vi "IQA.vi"() -> ()   [LabVIEW 2017]
uses:
  Sub VIs/Control/State machine.ctl
  <vilib>/Utility/miscctls.llb/LVPointTypeDef.ctl
  <vilib>/addons/database/Connection.llb/Conn ObjectReference.ctl
  5081ad37-31e8-4bc8-bbee-fac5e5d8bad7.vi
  <vilib>/Array/Sort 2D Array - Pop Stack.vi
  <vilib>/Array/Sort 2D Array - Push Stack.vi
  <vilib>/addons/database/Connection.llb/DB Tools Open Connec (Path).vi
  <vilib>/addons/database/Connection.llb/Conn Execute.vi
  <vilib>/addons/database/Recordset.llb/Rec Fetch Recordset Data (R).vi
  <vilib>/addons/database/Recordset.llb/Rec Destroy - Connection.vi
  <vilib>/addons/database/_DB Variant To Data/Database Variant To Data.xnode
  <vilib>/Utility/config.llb/NI_LVConfig.lvlib
  <vilib>/addons/database/NI_Database_API.lvlib
panel:
  out "local":T1
  out "server":T1
  in  "Search":string(combo)
  in  "IQA Check":bool
  in  "Refresh":bool
  in  "Invoice CODE":string(combo)
  out "Invoice Date":timestamp format="%<%d/%m/%Y>T"
  out "Table":string[][](table)
  # "IQA HISTORY"
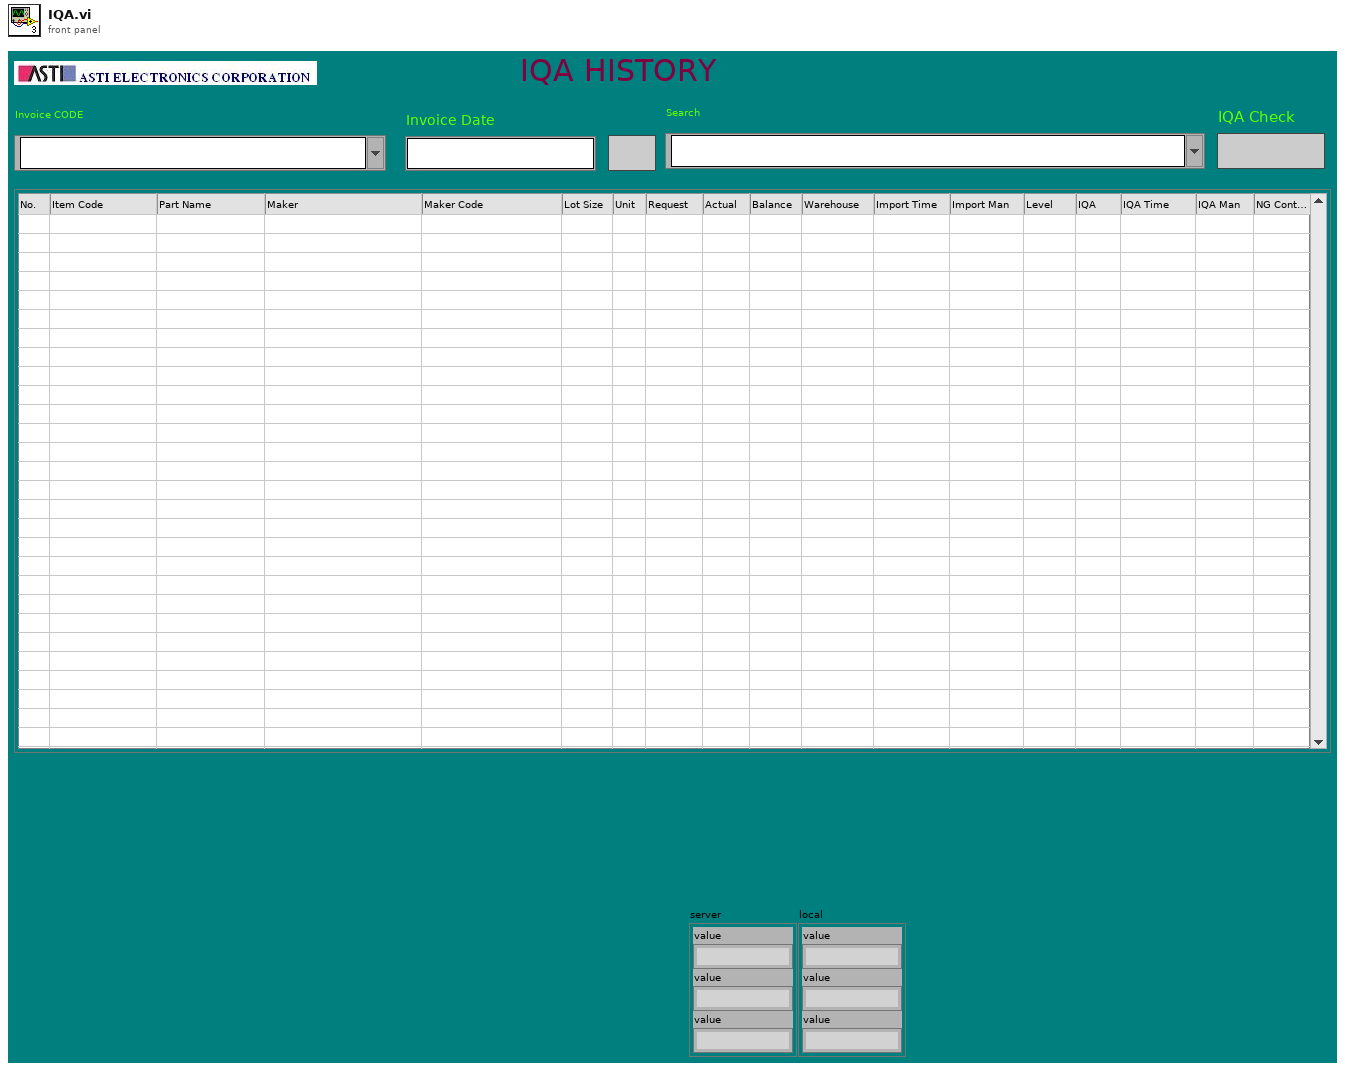
[diagram p1: front panel]
types:
  T1 = cluster{"value":string, "value":string, "value":string}
  T2 = typedef "NI_Database_API.lvlib/Conn ObjectReference.ctl" = refnum<k1>
  T3 = typedef "LVPointTypeDef.ctl" = cluster{"Horizontal":i16, "Vertical":i16}
  T4 = typedef "State machine.ctl" = enum16{"Licence check", "Initial", "Log in", "Creat Config file", "Network setting", "Creat database 1", "Creat database 2", "Creat database 3", "Transfer", "Begin", "Exit"}
  T5 = typedef "NI_LVConfig.lvlib/Config Data RefNum.ctl" = refnum<k1>
  T6 = typedef "NI_Database_API.lvlib/Rec ObjectReference.ctl" = refnum<k1>
  T7 = cluster{"[0]":string, "[1]":string, "[2]":string, "[3]":string, "[4]":string, "[5]":string, "[6]":string, "[7]":string, "[8]":string, "[9]":string, "[10]":string, "[11]":string, "[12]":string, "[13]":string, "[14]":string, "[15]":string}
  T8 = cluster{"[0]":string, "[1]":string, "[2]":string, "[3]":string, "[4]":string, "[5]":string, "[6]":string, "[7]":string, "[8]":string, "[9]":string, "[10]":string, "[11]":string, "[12]":string, "[13]":string, "[14]":string, "[15]":string}[]
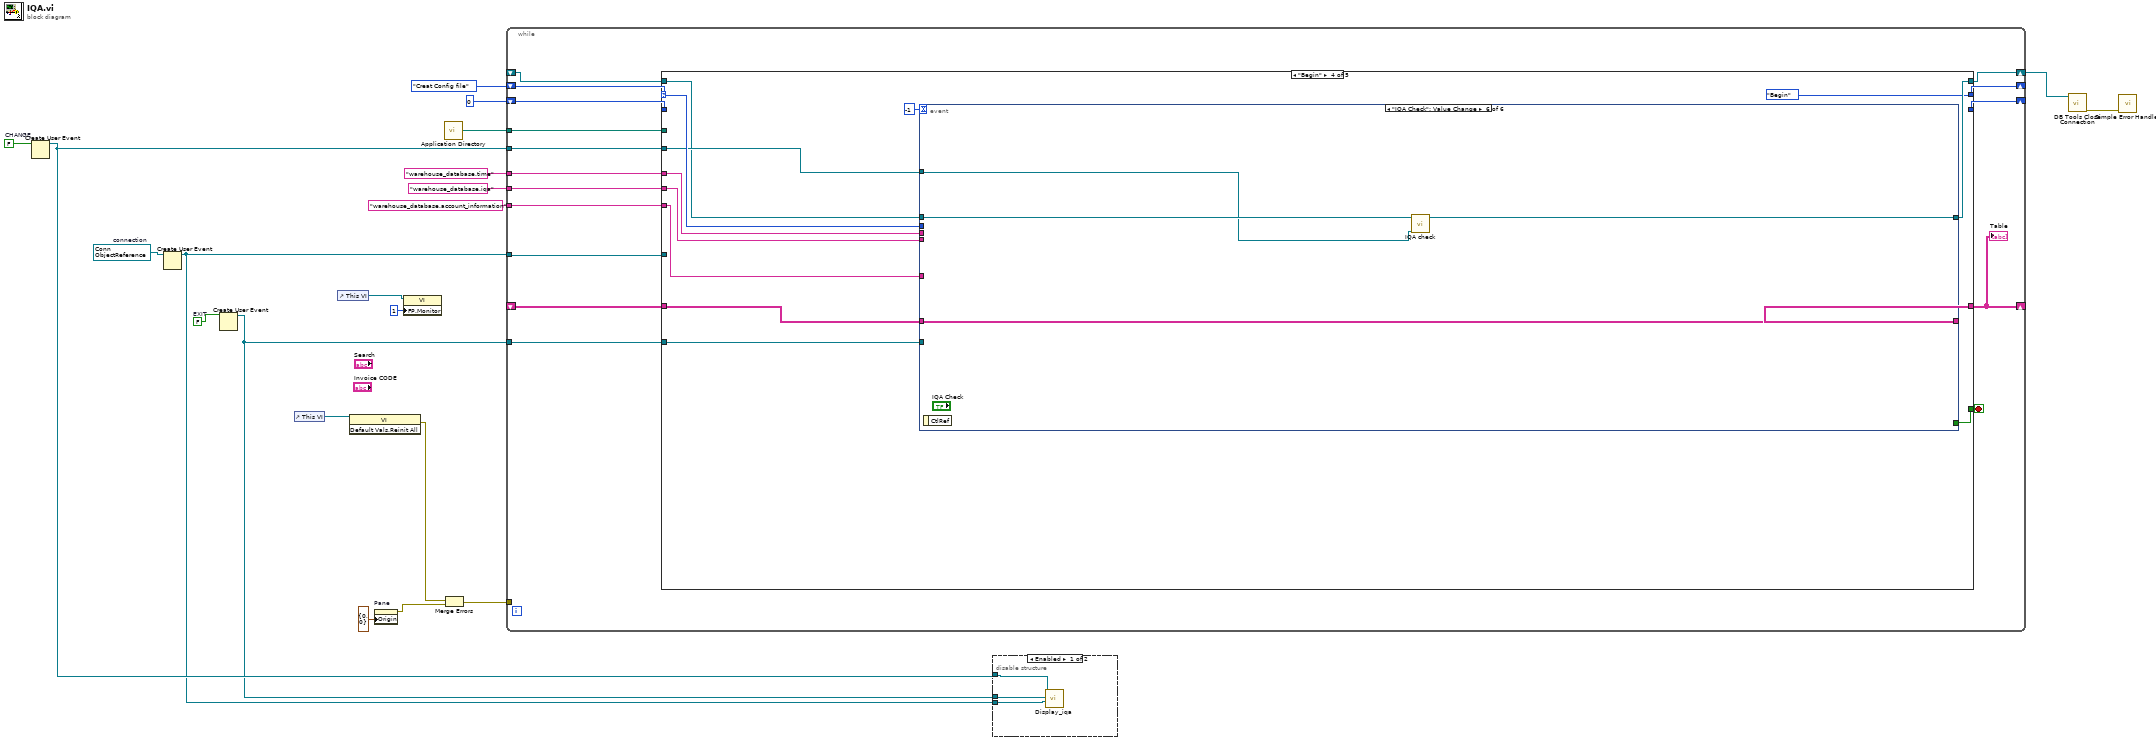
[diagram p0: block diagram]
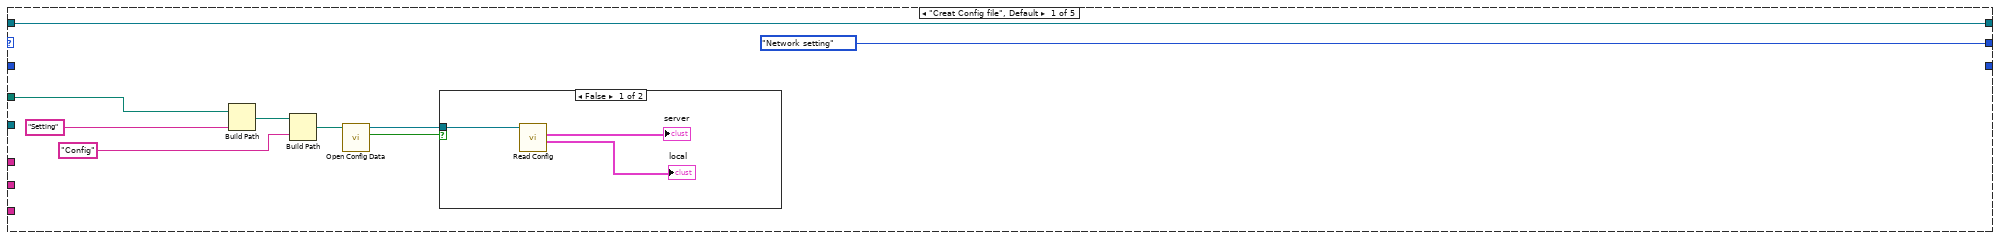
[diagram p3: hidden frame]
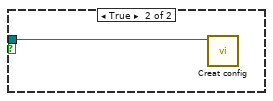
[diagram p4: hidden frame]
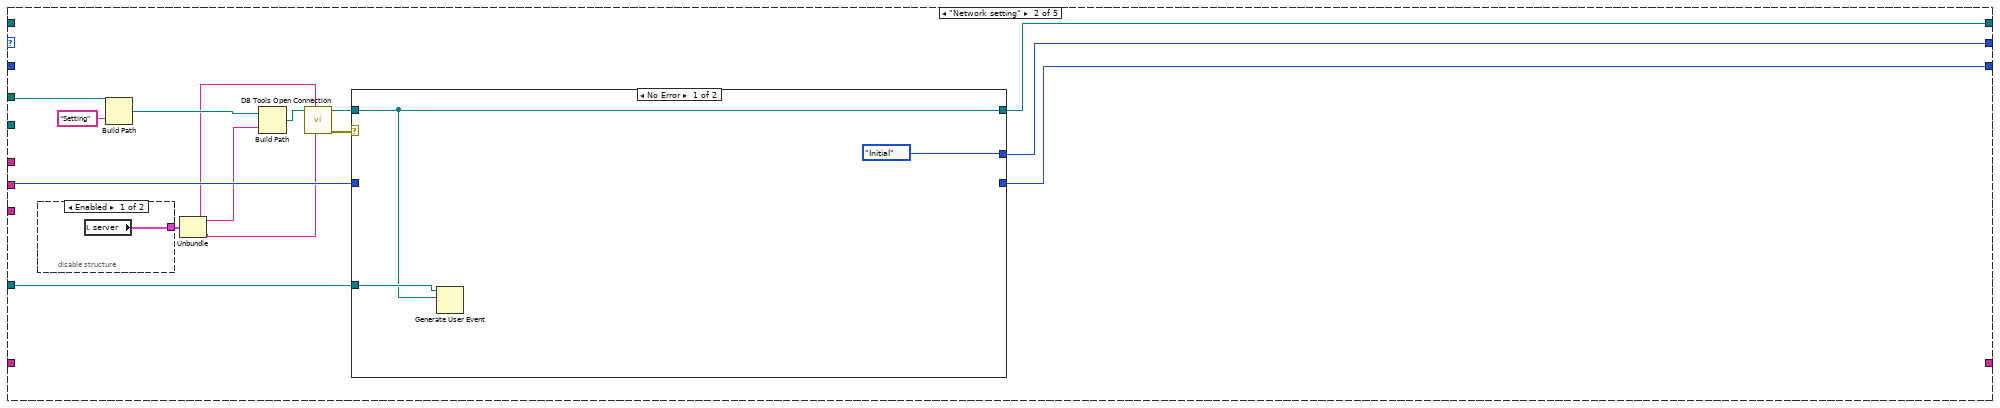
[diagram p5: hidden frame]
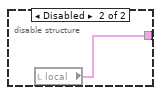
[diagram p6: hidden frame]
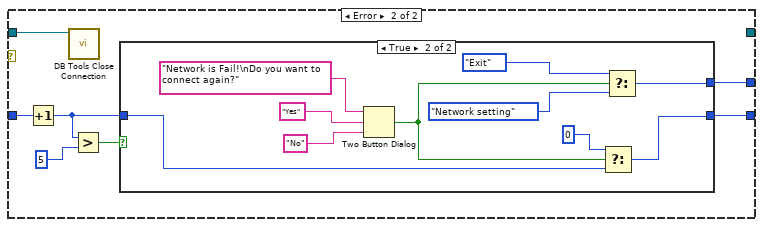
[diagram p7: hidden frame]
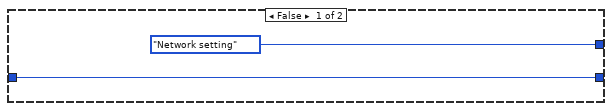
[diagram p8: hidden frame]
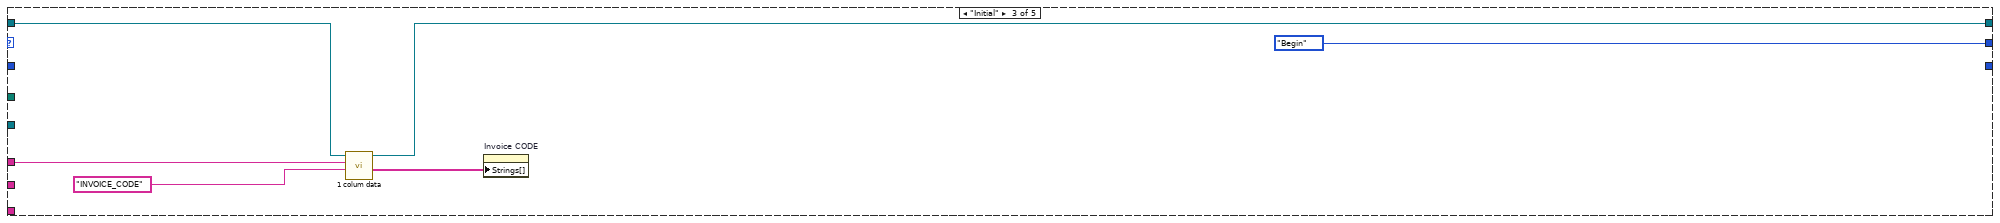
[diagram p9: hidden frame]
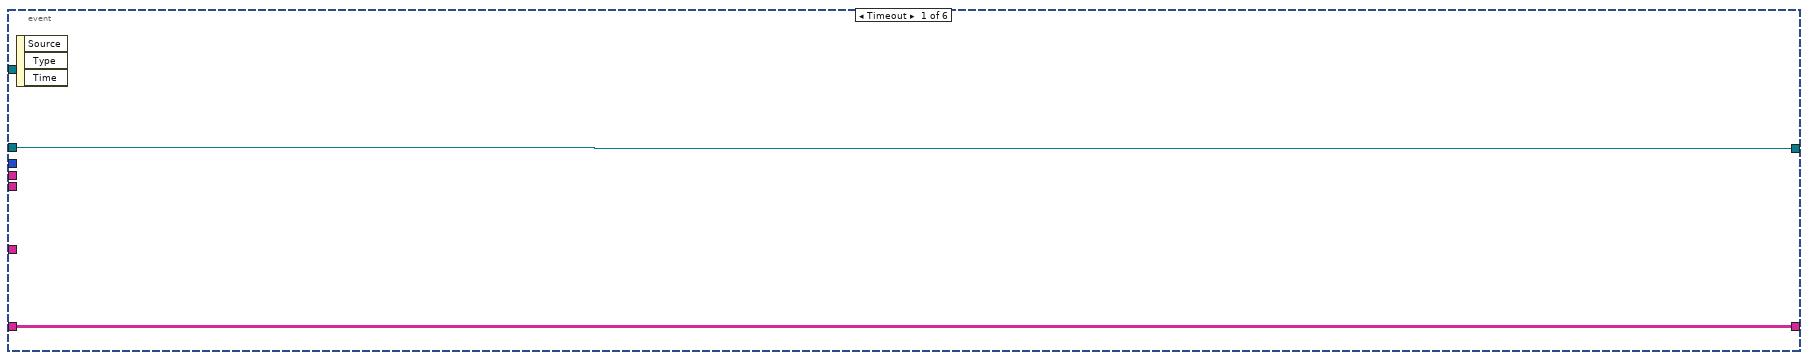
[diagram p10: hidden frame]
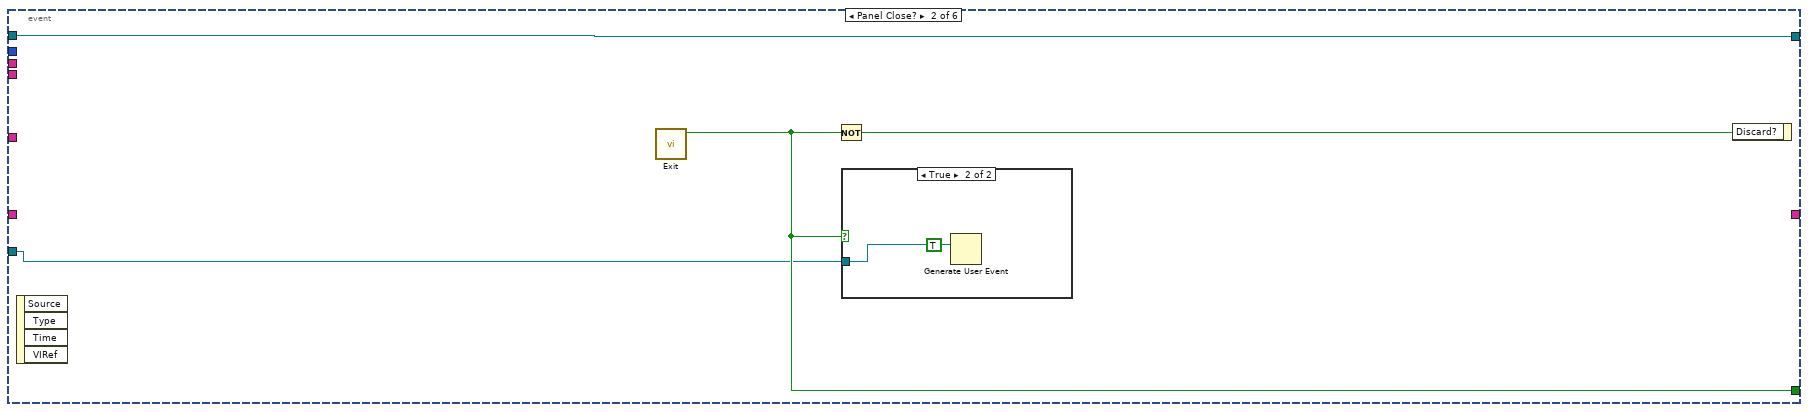
[diagram p11: hidden frame]
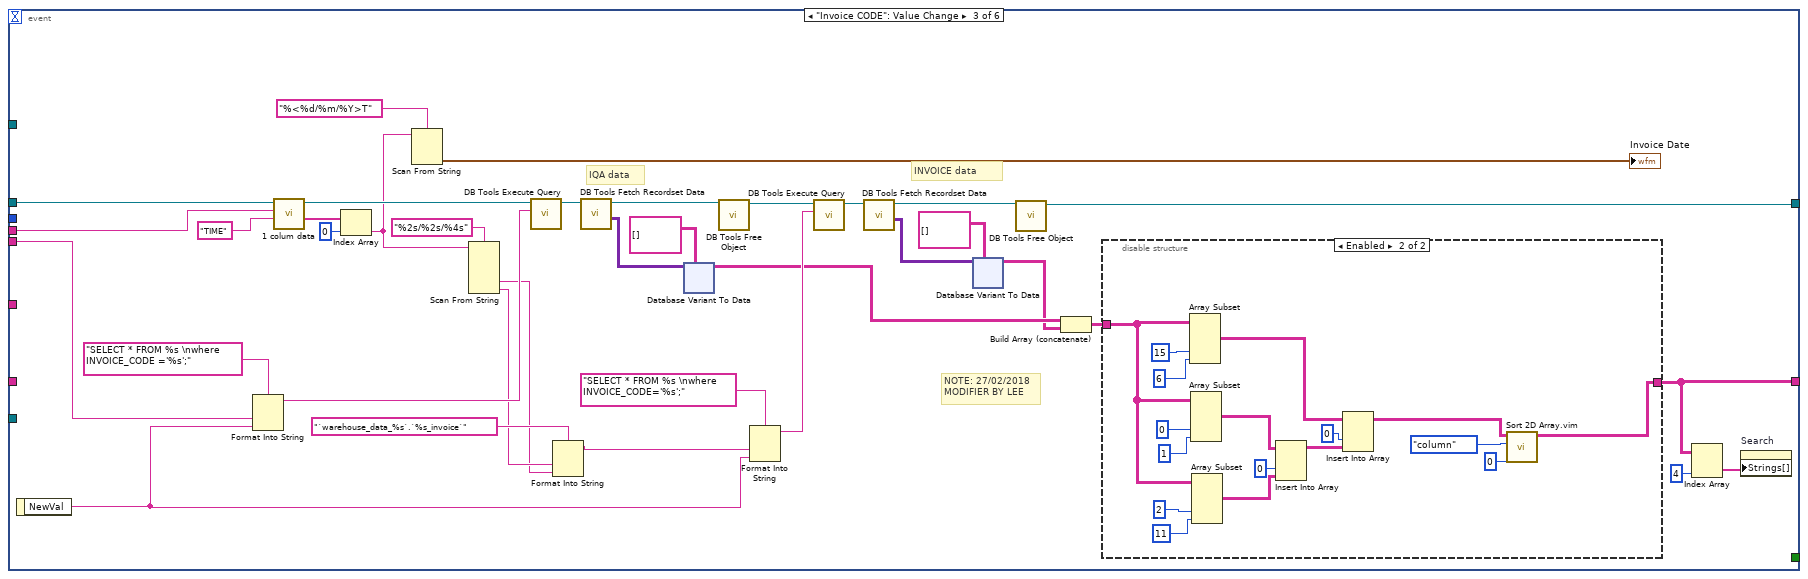
[diagram p13: hidden frame]
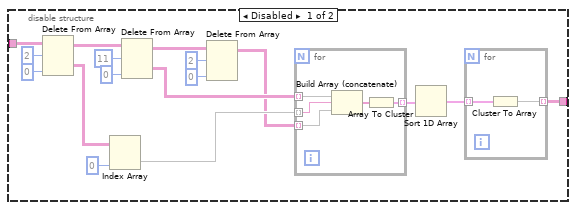
[diagram p14: hidden frame]
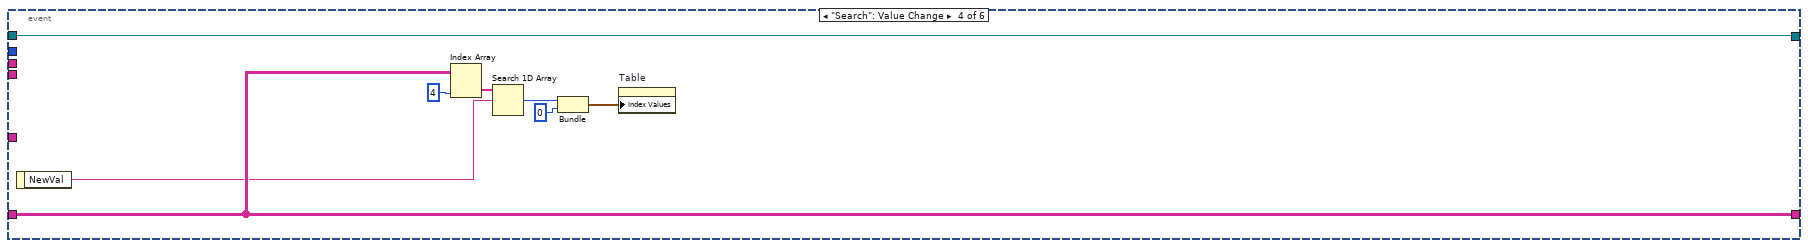
[diagram p15: hidden frame]
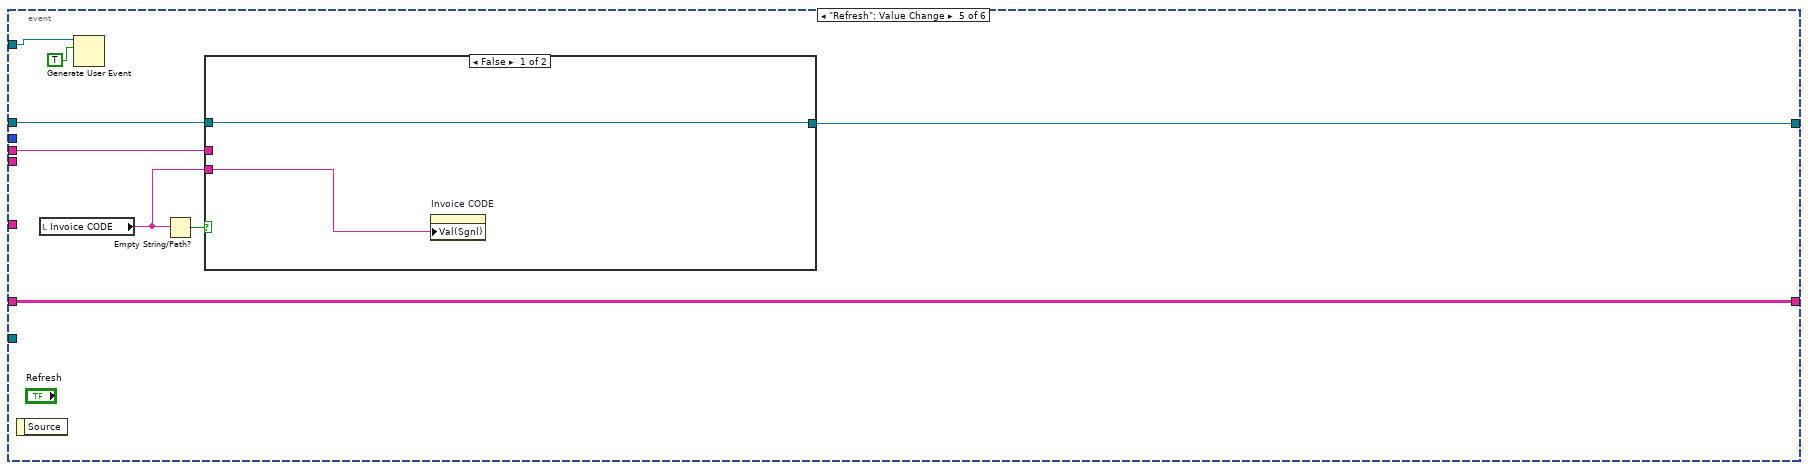
[diagram p16: hidden frame]
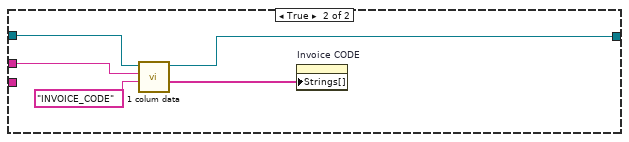
[diagram p17: hidden frame]
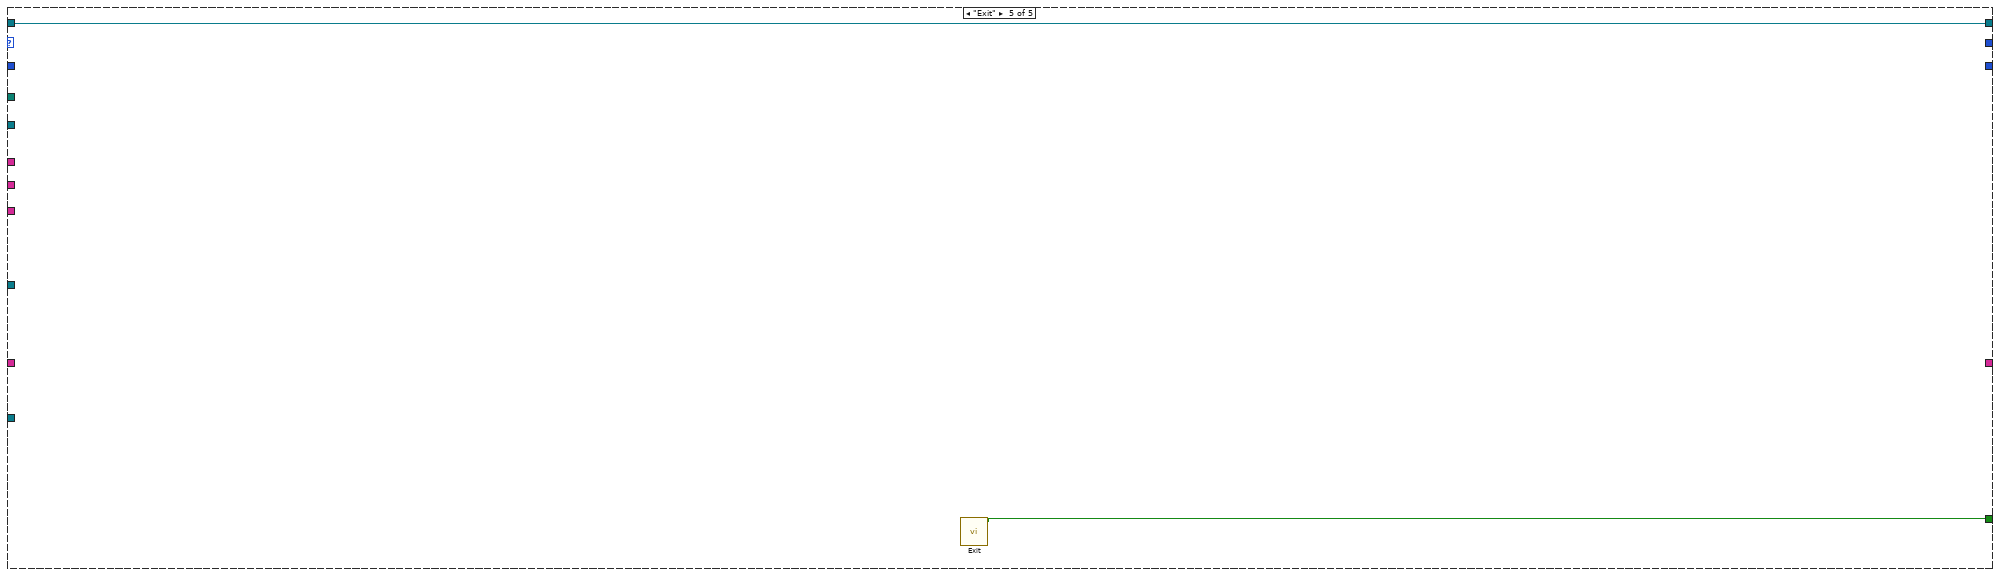
[diagram p18: hidden frame]
diagram:
  w1 = T2 refnum items=["Connection"]  # connection
  w4 = FALSE  # EXIT
  w6 = FALSE  # CHANGE
  n1 = Create User Event(user event datatype=w6) -> (user event=w5:refnum<user-event>)  [unwired: 1 in, 1 out]
  n2 = Create User Event(user event datatype=w1) -> (user event=w2:refnum<user-event>)  [unwired: 1 in, 1 out]
  n3 = Create User Event(user event datatype=w4) -> (user event=w3:refnum<user-event>)  [unwired: 1 in, 1 out]
  n4 = control-ref of="This VI"() -> (w16:refnum<vi>)
  n5 = control-ref of="This VI"() -> (w8:refnum<vi>)
  n6 = invoke class="VI" method="Default Vals.Reinit All"(reference=w16) -> (error out=w14:errorcluster)  [unwired: 2 in, 2 out]
  n7 = property on="Pane" class="Pane"("Origin"=T3 {"Horizontal"=0, "Vertical"=0}) -> (error out=w13:errorcluster)  [unwired: 2 in, 1 out]
  n8 = property class="VI"(reference=w8, "FP.Monitor"=u16 1 ("Front Panel Window:Monitor")) -> ()  [unwired: 1 in, 2 out]
  n9 = call <vilib>:"Application Directory.vi"() -> ("Application Directory"=w20:path)
  n10 = Merge Errors(w14, w13) -> (w12:errorcluster)
  n11 = while {
    shift-right: [w34] -> _
    shift-left: State_machine."Creat Config file" ("Enum") -> [w36]
    tunnel: w20 -> [w35]
    shift-right: [w33] -> w19
    shift-left: _ -> [w25]
    shift-right: [w31] -> _
    shift-left: 0 -> [w32]
    tunnel: w12 -> [_]
    tunnel: "warehouse_database.time" ("table") -> [w30]
    tunnel: "warehouse_database.iqa" ("table") -> [w29]
    tunnel: "warehouse_database.account_information" -> [w28]
    shift-right: [w26] -> _
    shift-left: _ -> [w27]
    tunnel: w5 -> [w24]
    tunnel: w3 -> [w23]
    tunnel: w2 -> [w22]
    stop <- w37 stop-if-true
    n12 = case shown="\"Begin\"" w36 {
      selector: w36 -> [_ _ _ w106 _]
      tunnel: [_ _ _ w108 w309] -> w37
      tunnel: w35 -> [w45 w59 _ _ _]
      tunnel: [State_machine."Network setting" ("Enum") w62 State_machine."Begin" ("Enum") State_machine."Begin" ("Enum") _] -> w34
      tunnel: [w38 w63 w93 w107 w310] -> w33
      tunnel: w25 -> [w38 _ w94 w96 w310]
      tunnel: w32 -> [_ w61 _ _ _]
      tunnel: [_ w60 _ _ _] -> w31
      tunnel: w30 -> [_ _ w90 w104 _]
      tunnel: w29 -> [_ _ _ w103 _]
      tunnel: w28 -> [_ _ _ w102 _]
      tunnel: [_ _ _ w101 _] -> w26
      tunnel: w27 -> [_ _ _ w100 _]
      tunnel: w24 -> [_ _ _ w99 _]
      tunnel: w23 -> [_ _ _ w98 _]
      tunnel: w22 -> [_ w51 _ _ _]
      frame "Creat Config file", Default {
        n13 = Build Path(base path=w45, name or relative path="Setting") -> (appended path=w43:path)
        n14 = Build Path(base path=w43, name or relative path="Config") -> (appended path=w41:path)
        n15 = call <vilib>:"Open Config Data.vi"("configuration file path"=w41) -> ("file created?"=w40:bool, "refnum"=w39:T5)  [unwired: 8 in, 1 out]
        n16 = case shown="False" w40 {
          tunnel: w39 -> [w49 w50]
          frame False {
            n17 = call "Read Config.vi"("Refnum in"=w49) -> ("local"=→"local":T1, "server"=→"server":T1)  [unwired: 9 in]
          }
          frame True {
            n18 = call "Creat config.vi"("Refnum in"=w50) -> ()  [unwired: 11 in]
          }
        }
      }
      frame "Network setting" {
        n19 = disable-structure shown="Enabled" {
          disable-tunnel: [w66 w67] -> w55
          frame Enabled {
            n20 = local read "server"() -> (w66:T1)
          }
          frame Disabled {
            n21 = local read "local"() -> (w67:T1)
          }
        }
        n22 = Build Path(base path=w59, name or relative path="Setting") -> (appended path=w56:path)
        n23 = Unbundle(w55) -> ("value"=w54:string, "value"=w53:string, "value"=w52:string)
        n24 = Build Path(base path=w56, name or relative path=w54) -> (appended path=w57:path)
        n25 = call-poly <vilib>:"DB Tools Open Connection.vi"("password"=w52, "userID"=w53, "connection information"=w57) -> ("error out"=w65:errorcluster, "connection reference"=w64:T2)  [unwired: 5 in]
        n26 = case shown="No Error" w65 {
          tunnel: w64 -> [w68 w77]
          tunnel: [w68 _] -> w63
          tunnel: [State_machine."Initial" ("Enum") w73] -> w62
          tunnel: w61 -> [_ w76]
          tunnel: [_ w72] -> w60
          tunnel: w51 -> [w69 _]
          frame No Error {
            n27 = Generate User Event(user event=w69, event data cluster=w68) -> ()  [unwired: 2 in, 2 out]
          }
          frame Error {
            n28 = Increment(x=w76) -> (x+1=w71:i32)
            n29 = call <vilib>:"DB Tools Close Connection.vi"("connection reference"=w77) -> ()  [unwired: 6 in, 1 out]
            n30 = Greater?(x=w71, y=5) -> (0:w74:bool)
            n31 = case shown="True" w74 {
              tunnel: [State_machine."Network setting" ("Enum") w84] -> w73
              tunnel: [w78 w81] -> w72
              tunnel: w71 -> [w78 w82]
              frame False {
              }
              frame True {
                n32 = Two Button Dialog(message="Network is Fail!\nDo you want to connect again?", 1:"No" ("F button name (\"Cancel\")"), 2:"Yes" ("T button name (\"OK\")")) -> (T button?=w83:bool)
                n33 = Select(t=0, s=w83, f=w82) -> (s? t:f=w81:i32)
                n34 = Select(t=State_machine."Exit" ("Enum"), s=w83, f=State_machine."Network setting" ("Enum")) -> (s? t:f=w84:T4)
              }
            }
          }
        }
      }
      frame "Initial" {
        n35 = call "1 colum data.vi"("column"="INVOICE_CODE" ("String"), "table"=w90, "Refnum in"=w94) -> ("data"=w91:string[], "Refnum out"=w93:T2)  [unwired: 6 in, 1 out]
        n36 = property on="Invoice CODE" class="CmbBox"("Strings[]"=w91) -> ()  [unwired: 2 in, 2 out]
      }
      frame "Begin" {
        n37 = event shown="[5] \"IQA Check\": Value Change" {
          selector: _ -> [_ _ _ _ _ _]
          dyn-events: _ -> [_ _ _ _ _ _]
          timeout: -1 -> [_ _ _ _ _ _]
          tunnel: [_ w112 _ _ _ _] -> w108
          tunnel: w96 -> [w110 w113 w152 w282 w290 w308]
          tunnel: [w110 w113 w136 w282 w297 w307] -> w107
          tunnel: w106 -> [_ _ _ _ _ _]
          tunnel: w104 -> [_ _ w151 _ w296 _]
          tunnel: w103 -> [_ _ w141 _ _ _]
          tunnel: w102 -> [_ _ _ _ _ _]
          tunnel: [w109 _ w123 w284 w293 w306] -> w101
          tunnel: w100 -> [w109 _ _ w284 w293 w306]
          tunnel: w99 -> [_ _ _ _ w292 w305]
          tunnel: w98 -> [_ w111 _ _ _ _]
          event Timeout {
            n38 = event-data() -> ()  [unwired: 1 in, 3 out]
          }
          event Panel Close? {
            n39 = event-data() -> ()  [unwired: 1 in, 4 out]
            n40 = call "Exit.vi"() -> ("T button?"=w112:bool)  [unwired: 11 in]
            n41 = Not(x=w112) -> (.not. x?=w114:bool)
            n42 = case shown="True" w112 {
              tunnel: w111 -> [_ w116]
              frame False {
              }
              frame True {
                n43 = Generate User Event(user event=w116, event data cluster=TRUE ("event data")) -> ()  [unwired: 2 in, 2 out]
              }
            }
            n44 = event-data("Discard?"=w114) -> ()  [unwired: 1 in, 1 out]
          }
          event "Invoice CODE": Value Change {
            # "NOTE: 27/02/2018\nMODIFIER BY LEE"
            # "INVOICE data"
            # "IQA data"
            n45 = event-data() -> ("NewVal"=w133:string)  [unwired: 1 in]
            n46 = Format Into String(format string="SELECT * FROM %s \nwhere INVOICE_CODE ='%s';", w141, w133) -> (resulting string=w140:string)  [unwired: 2 in, 1 out]
            n47 = call "1 colum data.vi"("column"="TIME", "table"=w151, "Refnum in"=w152) -> ("data"=w149:string[], "Refnum out"=w146:T2)  [unwired: 6 in, 1 out]
            n48 = Index Array(array=w149, index=0) -> (element=w126:string)
            n49 = Scan From String(format string="%<%d/%m/%Y>T", input string=w126) -> (output 1=→"Invoice Date":timestamp)  [unwired: 3 in, 3 out]
            n50 = Scan From String(format string="%2s/%2s/%4s", input string=w126) -> (output 2=w118:string, output 3=w119:string)  [unwired: 6 in, 3 out]
            n51 = call-poly <vilib>:"DB Tools Execute Query.vi"("SQL query"=w140, "connection reference"=w146) -> ("recordset reference"=w145:T6)  [unwired: 6 in, 1 out]
            n52 = Format Into String(format string="`warehouse_data_%s`.`%s_invoice`" ("string"), w119, w118) -> (resulting string=w117:string)  [unwired: 2 in, 1 out]
            n53 = call-poly <vilib>:"DB Tools Fetch Recordset Data.vi"("recordset reference"=w145) -> ("recordset data"=w143:variant[][], "recordset reference out"=w144:T6)  [unwired: 4 in, 1 out]
            n54 = xnode "Database Variant To Data"("database variant"=w143, "type"=string[][] []) -> ("data"=w129:string[][])  [unwired: 1 in, 1 out]
            n55 = call-poly <vilib>:"DB Tools Free Object.vi"("recordset reference"=w144) -> ("connection reference"=w137:T2)  [unwired: 9 in, 1 out]
            n56 = Format Into String(format string="SELECT * FROM %s \nwhere INVOICE_CODE='%s';", w117, w133) -> (resulting string=w132:string)  [unwired: 2 in, 1 out]
            n57 = call-poly <vilib>:"DB Tools Execute Query.vi"("SQL query"=w132, "connection reference"=w137) -> ("recordset reference"=w138:T6)  [unwired: 6 in, 1 out]
            n58 = call-poly <vilib>:"DB Tools Fetch Recordset Data.vi"("recordset reference"=w138) -> ("recordset data"=w130:variant[][], "recordset reference out"=w139:T6)  [unwired: 4 in, 1 out]
            n59 = xnode "Database Variant To Data"("database variant"=w130, "type"=string[][] []) -> ("data"=w128:string[][])  [unwired: 1 in, 1 out]
            n60 = call-poly <vilib>:"DB Tools Free Object.vi"("recordset reference"=w139) -> ("connection reference"=w136:T2)  [unwired: 9 in, 1 out]
            n61 = Build Array (concatenate)(w129, w128) -> (w127:string[][])
            n62 = disable-structure shown="Enabled" {
              disable-tunnel: w127 -> [w169 w181]
              disable-tunnel: [w153 w193] -> w123
              frame Disabled {
                n63 = Delete From Array(array=w169, length=2, index (col)=0 ("disabled index (col)")) -> (deleted portion=w160:string[][], array with subset deleted=w166:string[][])  [unwired: 1 in]
                n64 = Index Array(array=w160, index (col)=0 ("disabled index (col)")) -> (element=w157:string[])  [unwired: 1 in]
                n65 = Delete From Array(array=w166, length=11, index (col)=0 ("disabled index (col)")) -> (deleted portion=w158:string[][], array with subset deleted=w161:string[][])  [unwired: 1 in]
                n66 = Delete From Array(array=w161, length=2, index (col)=0 ("disabled index (col)")) -> (array with subset deleted=w156:string[][])  [unwired: 1 in, 1 out]
                n67 = for {
                  tunnel: w158 -> [w176] mode=indexing
                  tunnel: w157 -> [w175] mode=indexing
                  tunnel: w156 -> [w174] mode=indexing
                  tunnel: [w172] -> w155 mode=indexing
                  n68 = Build Array (concatenate)(w176, w175, w174) -> (w173:string[])
                  n69 = Array To Cluster(array=w173) -> (cluster=w172:T7)
                }
                n70 = Sort 1D Array(array=w155) -> (sorted array=w154:T8)
                n71 = for {
                  tunnel: w154 -> [w171] mode=indexing
                  tunnel: [w170] -> w153 mode=indexing
                  n72 = Cluster To Array(cluster=w171) -> (array=w170:string[])
                }
              }
              frame Enabled {
                n73 = Array Subset(array=w181, index (col)=15 ("index"), length (col)=6 ("length")) -> (w179:string[][])  [unwired: 2 in]
                n74 = Array Subset(array=w181, index (col)=0 ("index"), length (col)=1 ("length")) -> (w186:string[][])  [unwired: 2 in]
                n75 = Array Subset(array=w181, index (col)=2 ("index"), length (col)=11 ("length")) -> (w185:string[][])  [unwired: 2 in]
                n76 = Insert Into Array(array=w186, index (col)=0 ("disabled index (col)"), new element=w185) -> (w178:string[][])  [unwired: 1 in]
                n77 = Insert Into Array(array=w179, index (col)=0 ("disabled index (col)"), new element=w178) -> (w177:string[][])  [unwired: 1 in]
                n78 = call "Sort 2D Array.vim"("index"=0, "dimension to index (column)"=enum16{"column", "row"}."column", "2D array"=w177) -> ("sorted 2D array"=w193:string[][])  [unwired: 7 in, 1 out]
              }
            }
            n79 = Index Array(array=w123, index (col)=4 ("disabled index (col)")) -> (element=w121:string[])  [unwired: 1 in]
            n80 = property on="Search" class="CmbBox"("Strings[]"=w121) -> ()  [unwired: 2 in, 2 out]
          }
          event "Search": Value Change {
            n81 = event-data() -> ("NewVal"=w283:string)  [unwired: 1 in]
            n82 = Index Array(array=w284, index (col)=4 ("disabled index (col)")) -> (element=w286:string[])  [unwired: 1 in]
            n83 = Search 1D Array(1D array=w286, element=w283) -> (index of element=w289:i32)  [unwired: 1 in]
            n84 = Bundle("index of element"=w289, 0) -> (w288:cluster{"index of element":i32, i32})  [unwired: 1 in]
            n85 = property on="Table" class="Tbl (strict)"("Index Values"=w288) -> ()  [unwired: 2 in, 2 out]
          }
          event "Refresh": Value Change {
            n86 = event-data() -> ()  [unwired: 1 in, 1 out]
            n87 = local read "Invoice CODE"() -> (w294:string)
            n88 = Generate User Event(user event=w292, event data cluster=TRUE ("event data")) -> ()  [unwired: 2 in, 2 out]
            n89 = Empty String/Path?(string/path=w294) -> (empty?=w295:bool)
            n90 = case shown="False" w295 {
              tunnel: w290 -> [w299 w302]
              tunnel: [w299 w301] -> w297
              tunnel: w296 -> [_ w300]
              tunnel: w294 -> [w298 _]
              frame False {
                n91 = property on="Invoice CODE" class="CmbBox"("Val(Sgnl)"=w298) -> ()  [unwired: 2 in, 2 out]
              }
              frame True {
                n92 = call "1 colum data.vi"("column"="INVOICE_CODE" ("String"), "table"=w300, "Refnum in"=w302) -> ("data"=w303:string[], "Refnum out"=w301:T2)  [unwired: 6 in, 1 out]
                n93 = property on="Invoice CODE" class="CmbBox"("Strings[]"=w303) -> ()  [unwired: 2 in, 2 out]
              }
            }
          }
          event "IQA Check": Value Change {
            n94 = event-data() -> ()  [unwired: 1 in, 1 out]
            n95 = call "IQA check.vi"("CHANGE"=w305, "connection in"=w308) -> ("connection out"=w307:T2)  [unwired: 9 in]
          }
        }
      }
      frame "Exit" {
        n96 = call "Exit.vi"() -> ("T button?"=w309:bool)  [unwired: 11 in]
      }
    }
    "Table" <- w26
  }
  n97 = disable-structure shown="Enabled" {
    disable-tunnel: w5 -> [w312 _]
    disable-tunnel: w3 -> [w313 _]
    disable-tunnel: w2 -> [w311 _]
    frame Enabled {
      n98 = call "Display_iqa.vi"("connection"=w311, "EXIT"=w313, "CHANGE"=w312) -> ()  [unwired: 9 in]
    }
    frame Disabled {
    }
  }
  n99 = call <vilib>:"DB Tools Close Connection.vi"("connection reference"=w19) -> ("error out"=w17:errorcluster)  [unwired: 6 in]
  n100 = call <vilib>:"Simple Error Handler.vi"("error in (no error)"=w17) -> ()  [unwired: 4 in, 5 out]
